vi "DateTime.vi"() -> ()   [LabVIEW 2020]
uses:
  <vilib>/addons/database/Auxilliary.llb/DB Tools Format Datetime String (Time Stamp).vi
  <vilib>/addons/database/_DB Variant To Data/Database Variant To Data.xnode
  <vilib>/addons/database/NI_Database_API.lvlib
panel:
  out "DateTime2 from DB":timestamp
  out "DateTime1 from DB":timestamp
  in  "error in (no error)":errorcluster
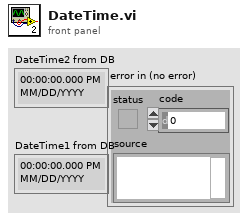
[diagram p1: front panel]
types:
  T1 = typedef "NI_Database_API.lvlib/Conn ObjectReference.ctl" = refnum<k1>
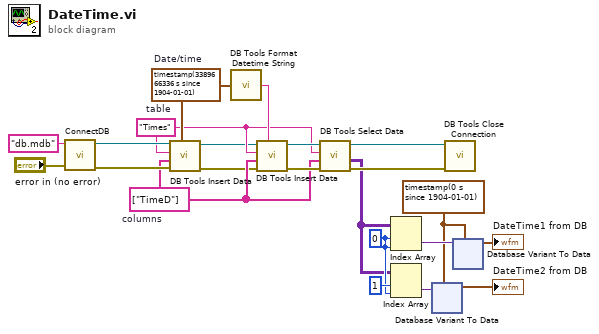
[diagram p0: block diagram]
diagram:
  w5 = 0 ("index (row)")
  w2 = timestamp(0 s since 1904-01-01)
  w18 = timestamp(3389666336.917968 s since 1904-01-01)  # Date/time
  w9 = string[] ["TimeD"]  # columns
  w13 = "Times"  # table
  n1 = call "ConnectDB.vi"("error in (no error)"="error in (no error)", "Filename"="db.mdb") -> ("error out"=w19:errorcluster, "DB Conn"=w20:T1)  [unwired: 8 in]
  n2 = call <vilib>:"DB Tools Insert Data.vi"("data"=w18, "error in (no error)"=w19, "columns"=w9, "table"=w13, "connection reference"=w20) -> ("error out"=w7:errorcluster, "connection reference out"=w8:T1)  [unwired: 5 in]
  n3 = call-poly <vilib>:"DB Tools Format Datetime String.vi"("time stamp"=w18) -> ("date/time string"=w17:string)
  n4 = call <vilib>:"DB Tools Insert Data.vi"("data"=w17, "error in (no error)"=w7, "columns"=w9, "table"=w13, "connection reference"=w8) -> ("error out"=w15:errorcluster, "connection reference out"=w14:T1)  [unwired: 5 in]
  n5 = call <vilib>:"DB Tools Select Data.vi"("error in (no error)"=w15, "columns"=w9, "table"=w13, "connection reference"=w14) -> ("error out"=w12:errorcluster, "data"=w4:variant[][], "connection reference out"=w11:T1)  [unwired: 2 in]
  n6 = Index Array(array=w4, index (row)=w5, index (col)=w5) -> (element=w16:variant)
  n7 = Index Array(array=w4, index (row)=1, index (col)=w5) -> (element=w3:variant)
  n8 = xnode "Database Variant To Data"("database variant"=w3, "type"=w2) -> ("data"=→"DateTime2 from DB":timestamp)  [unwired: 1 in, 1 out]
  n9 = call <vilib>:"DB Tools Close Connection.vi"("error in (no error)"=w12, "connection reference"=w11) -> ()  [unwired: 5 in, 1 out]
  n10 = xnode "Database Variant To Data"("database variant"=w16, "type"=w2) -> ("data"=→"DateTime1 from DB":timestamp)  [unwired: 1 in, 1 out]
